vi "Microscope.GetPublicEvents.vi"(8 "error in (no error)":errorcluster, 11 "Microscope":refnum<class "Microscope.lvclass">) -> (0 "error out":errorcluster, 2 "Microscope Public Events":T1, 3 "Microscope out":refnum<class "Microscope.lvclass">)   [LabVIEW 2015, in "Microscope.lvclass"]
doc: "---------------------------------------------------------------\nJKI State Machine Objects™\nhttp://jki.net/state-machine-objects/\nCopyright (C) 2005-2015, JKI <info@jki.net>\nALL RIGHTS RESERVEDJKI State Machine Objects (SMO) 1.0.0.5\nJKI - JKI\nCopyright (c) 2016, JKI"
uses:
  Microscope.lvclass
  Typedefs/PublicEvents--Cluster.ctl
  Typedefs/ValueChanged--EventData--Cluster.ctl
  Typedefs/PublicEvents--Microscope.Initialized.ctl
  Microscope.lvclass/Microscope.ctl
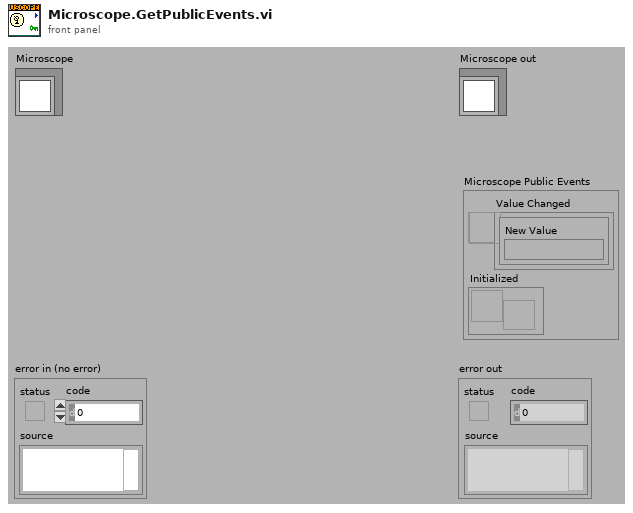
[diagram p1: front panel]
types:
  T1 = typedef "Microscope.lvclass/PublicEvents--Cluster.ctl" = cluster{"Value Changed":refnum<user-event>, "Initialized":refnum<user-event>}
  T2 = typedef "Microscope.lvclass/PrivateData--Ref.ctl" = refnum<data-value>
  T3 = typedef "Microscope.lvclass/PrivateData--Cluster.ctl" = cluster{"Public Events":T1, "Protected Events":T4, "Private Events":T5, "Dependencies":T6, "Configuration":T7}
  T4 = typedef "Microscope.lvclass/ProtectedEvents--Cluster.ctl" = cluster{"placeholder":refnum<user-event>}
  T5 = typedef "Microscope.lvclass/PrivateEvents--Cluster.ctl" = cluster{"New Value":refnum<user-event>, "Initialize":refnum<user-event>, "CaptureImageAtPosition":refnum<user-event>}
  T6 = typedef "Microscope.lvclass/Dependencies--Cluster.ctl" = cluster{"XYStage":refnum<class "XYStage.lvclass">, "Camera":refnum<class "Camera.lvclass">}
  T7 = typedef "Microscope.lvclass/Configuration--Cluster.ctl" = cluster{"XY Stage":string, "Camera":string, "image output folder":path, "filetype":string}
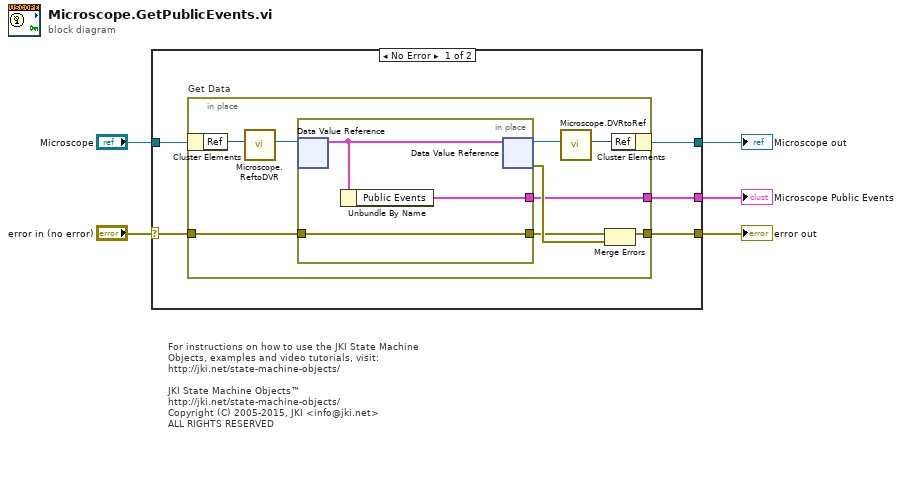
[diagram p0: block diagram]
diagram:
  # "For instructions on how to use the JKI State Machine Objects, examples and video tutorials, visit:\nhttp://jki.net/state-machine-objects/\n\nJKI State Machine Objects™\nhttp://jki.net/state-machine-objects/\nCopyright (C) 2005-2015, JKI <info@jki.net>\nALL RIGHTS RESERVED"
  n1 = case shown="No Error" "error in (no error)" {
    selector: "error in (no error)" -> [w9 w23]
    tunnel: "Microscope" -> [w10 w24]
    tunnel: [w8 w23] -> w4
    tunnel: [w6 w24] -> w3
    tunnel: [w7 _] -> w1
    frame No Error {
      n2 = in-place "Get Data" {
        in-place-border: w9 -> [w19]
        in-place-border: [w16] -> w8
        in-place-border: [w15] -> w7
        n3 = in-place-cluster #1(w10) -> ("Ref"=w14:u32)
        n4 = call "Microscope.ReftoDVR.vi"("Ref"=w14) -> ("Ref"=w13:T2)  [unwired: 10 in]
        n5 = in-place {
          in-place-border: w19 -> [w21]
          in-place-border: [w21] -> w17
          in-place-border: [w20] -> w15
          n6 = in-place-dvr #2(w13) -> (w22:T3)  [unwired: 1 out]
          n7 = Unbundle By Name(w22) -> ("Public Events"=w20:T1)
          n8 = in-place-dvr #2(w22) -> (w12:T2, w18:errorcluster)
        }
        n9 = call "Microscope.DVRtoRef.vi"("Ref"=w12) -> ("Ref"=w11:u32)  [unwired: 10 in]
        n10 = Merge Errors(w17, w18) -> (w16:errorcluster)
        n11 = in-place-cluster #1("Ref"=w11) -> (w6:refnum<class "Microscope.lvclass">)
      }
    }
    frame Error {
    }
  }
  "error out" <- w4
  "Microscope out" <- w3
  "Microscope Public Events" <- w1
